vi "init_cam_topLvl_v02.vi"(8 "error in":errorcluster, 9 "exposure (ms)":dbl=0.1 format="%#_13g", 10 "orig image":T3, 11 "cam info in":T1={"camera type"=enum."Qcam", "cam handle"=0, "data handle"=0, "cam size"=[]}) -> (0 "error out":errorcluster, 3 "cam info out":T1={"camera type"=enum."Qcam", "cam handle"=0, "data handle"=0, "cam size"=[]})   [LabVIEW 2015]
uses:
  <vilib>/vision/Image Controls.llb/IMAQ Image.ctl
  controls/cam_info.ctl
  controls/cam_type-v02.ctl
panel:
  # "init_cam"
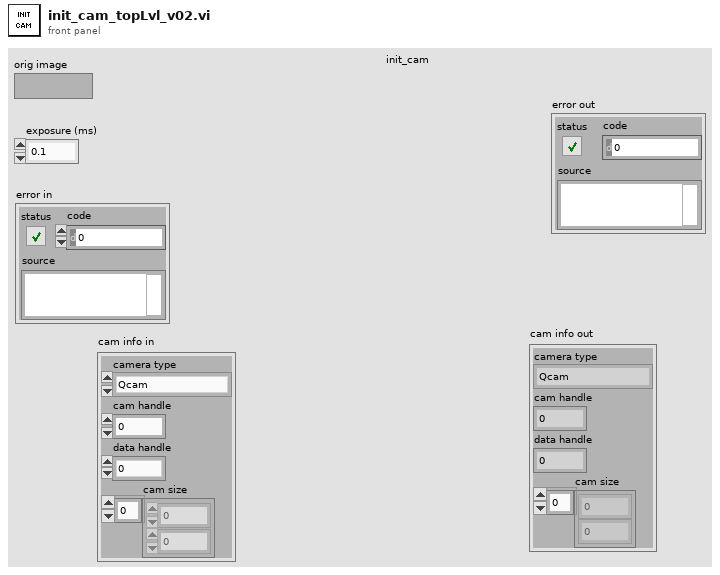
[diagram p1: front panel]
types:
  T1 = typedef "cam_info.ctl" = cluster{"camera type":T2, "cam handle":u32, "data handle":u32, "cam size":i32[]}
  T2 = typedef "cam_type-v02.ctl" = enum16{"HamamatsuORCA05G", "Qcam", "optiMOS"}
  T3 = typedef "IMAQ Image.ctl" = refnum<image>
  T4 = cluster{"acquire focus mode":u32, "exposure (ms)":dbl, i32, "Software accumulation":u32}
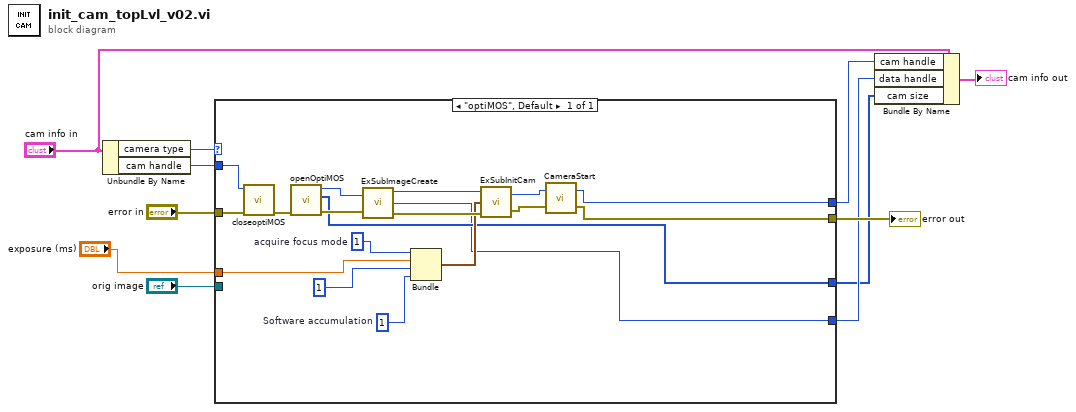
[diagram p0: block diagram]
diagram:
  n1 = Unbundle By Name("cam info in") -> ("camera type"=w8:T2, "cam handle"=w2:u32)
  n2 = case shown="\"optiMOS\", Default" w8 {
    tunnel: "orig image" -> [_]
    tunnel: [w19] -> w5
    tunnel: [w18] -> w10
    tunnel: "error in" -> [w14]
    tunnel: [w17] -> w3
    tunnel: [w16] -> w4
    tunnel: w2 -> [w15]
    tunnel: "exposure (ms)" -> [w12]
    frame "optiMOS", Default {
      w25 = u32 1  # acquire focus mode
      w23 = u32 1  # Software accumulation
      n3 = call "closeoptiMOS.vi"("error in (no error)"=w14, "Camera Handle"=w15) -> ("error out"=w13:errorcluster)  [unwired: 7 in]
      n4 = call "openOptiMOS.vi"("error in (no error)"=w13) -> ("error out"=w28:errorcluster, "cam size"=w17:i32[], "Camera Handle out"=w29:u32)  [unwired: 6 in]
      n5 = call "ExSubImageCreate.vi"("Camera Handle"=w29, "error in (no error)"=w28) -> ("Camera Handle"=w27:u32, "Data Handle"=w16:u32, "error out"=w26:errorcluster)
      n6 = Bundle("acquire focus mode"=w25, "exposure (ms)"=w12, 1, "Software accumulation"=w23) -> (w22:T4)  [unwired: 1 in]
      n7 = call "ExSubInitCam.vi"("error in (no error)"=w26, "Camera Information"=w22, "Camera Handle"=w27) -> ("error out"=w20:errorcluster, "Camera Handle"=w21:u32)
      n8 = call <userlib>:"CameraStart.vi"("error in"=w20, "Camera Handle"=w21) -> ("error out"=w18:errorcluster, "Camera Handle"=w19:u32)
    }
  }
  "error out" <- w10
  n9 = Bundle By Name(cluster="cam info in", "cam handle"=w5, "data handle"=w4, "cam size"=w3) -> (→"cam info out":T1)
